vi "CLD 14 Timer Application Solution.vi"() -> ()   [LabVIEW 2009]
doc: "CLD 14 Solution. This is a queued state machine using an array as the queue. The timer was adapted from CLD exercise three.\n\nThe Timer FGV is always running. Use time target equal to zero as the signal the timer is not \"active\""
uses:
  CLD 14 FGV Enum.ctl
  CLD 14 State Machine Enum.ctl
  CLD 14 CSV file enum.ctl
panel:
  out "Time Target (s)":dbl
  out "Elapsed Time (s)":dbl format="%#.2g"
  in  "Stop":bool
  in  "Pause":bool
  in  "cancel":bool
  in  "Start":bool
  in  "Error In":errorcluster
  out "Error Out":errorcluster
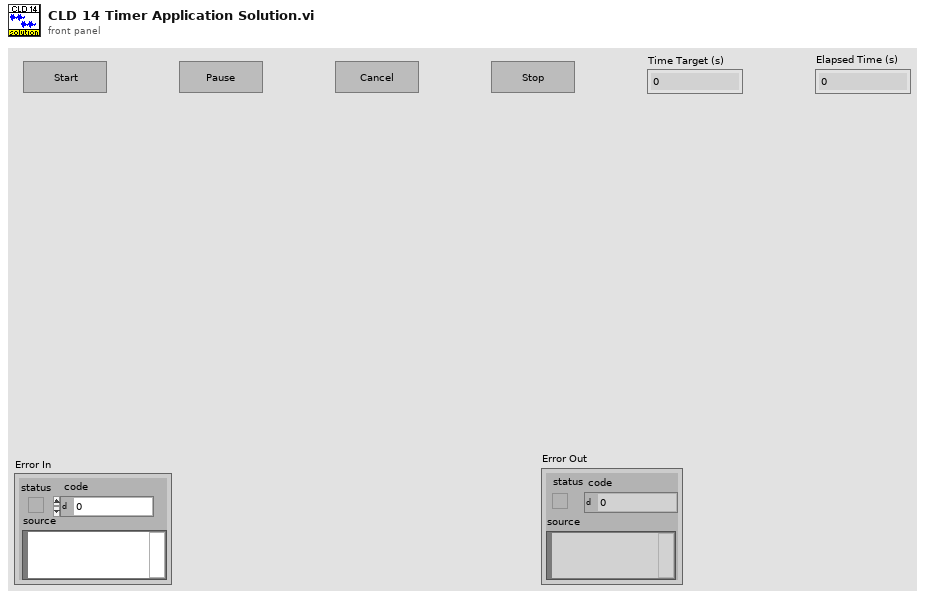
[diagram p1: front panel]
types:
  T1 = typedef "CLD 14 FGV Enum.ctl" = enum16{"Start Timer", "Read Time", "Pause", "UnPause"}
  T2 = typedef "CLD 14 State Machine Enum.ctl" = enum16{"Idle", "Initialize", "Run State", "Change Time", "CheckTime", "Start Time", "Pause", "UnPause"}
  T3 = typedef "CLD 14 CSV file enum.ctl" = enum16{"Read CSV", "Write CSV"}
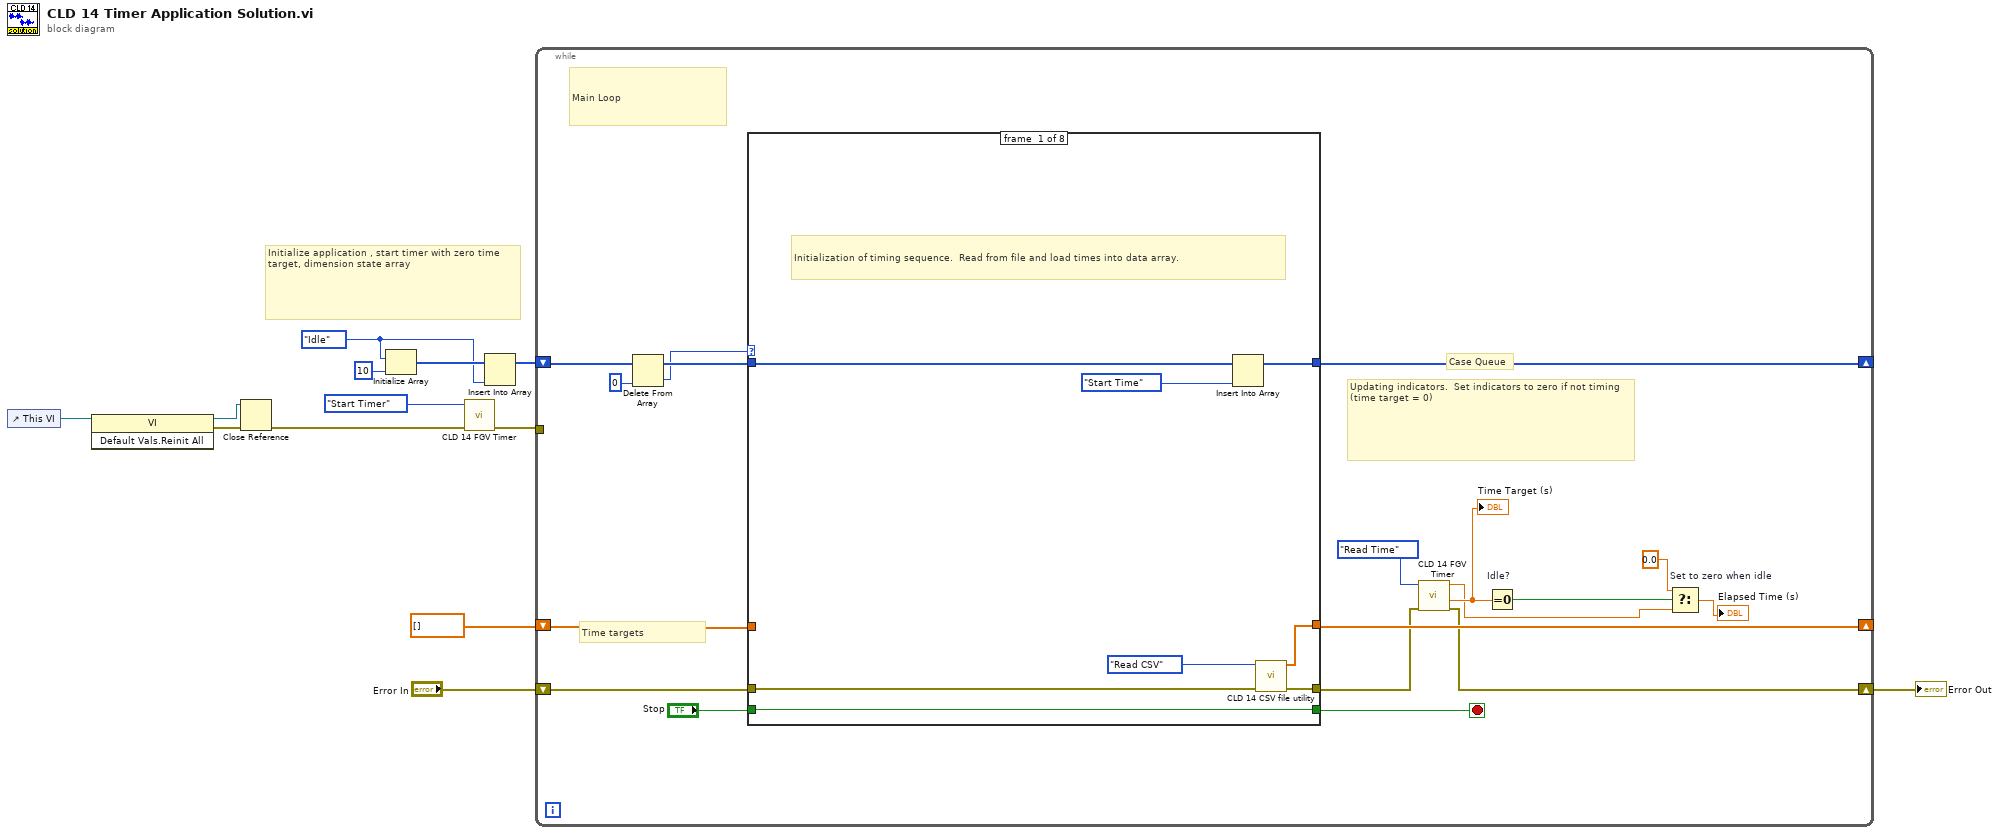
[diagram p0: block diagram]
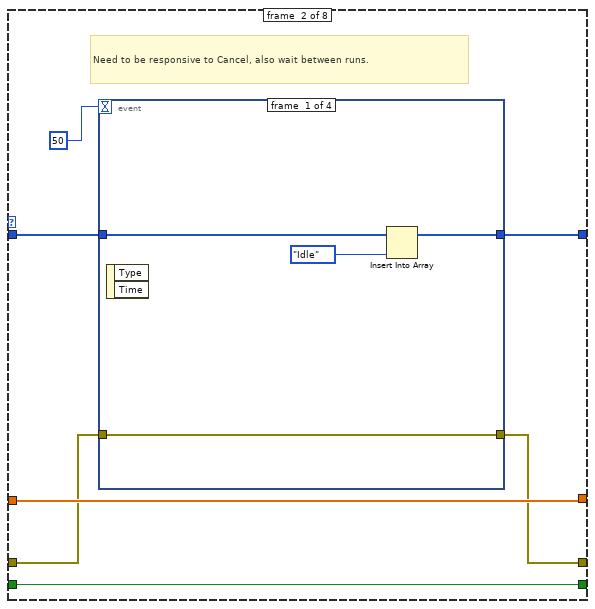
[diagram p2: hidden frame]
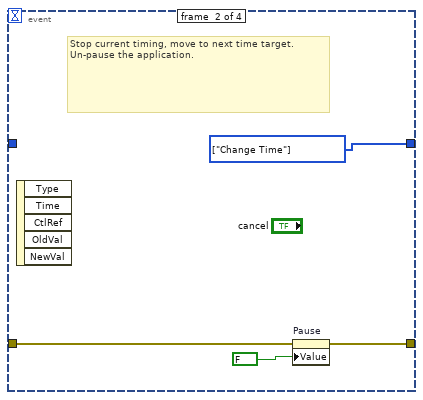
[diagram p3: hidden frame]
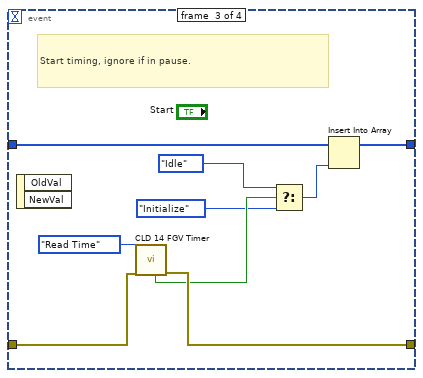
[diagram p4: hidden frame]
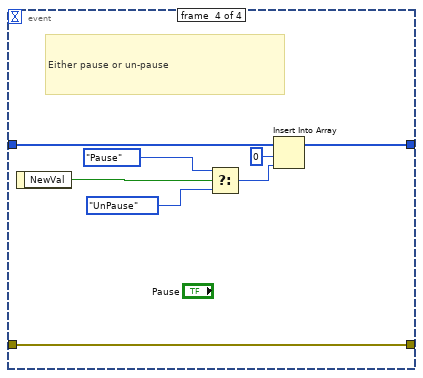
[diagram p5: hidden frame]
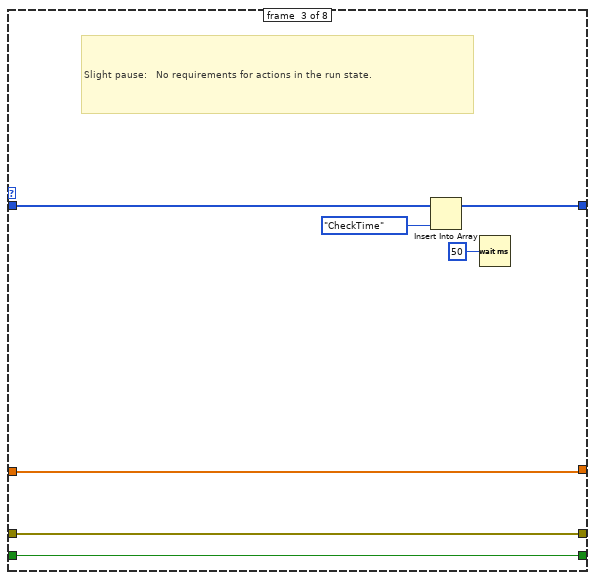
[diagram p6: hidden frame]
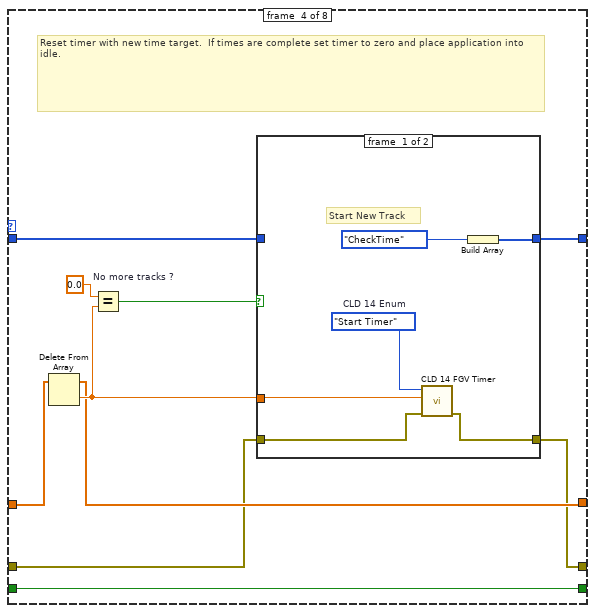
[diagram p7: hidden frame]
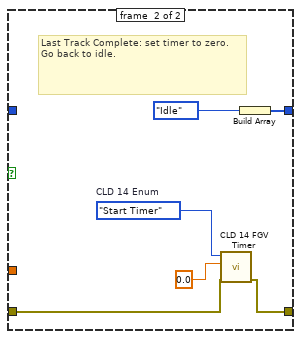
[diagram p8: hidden frame]
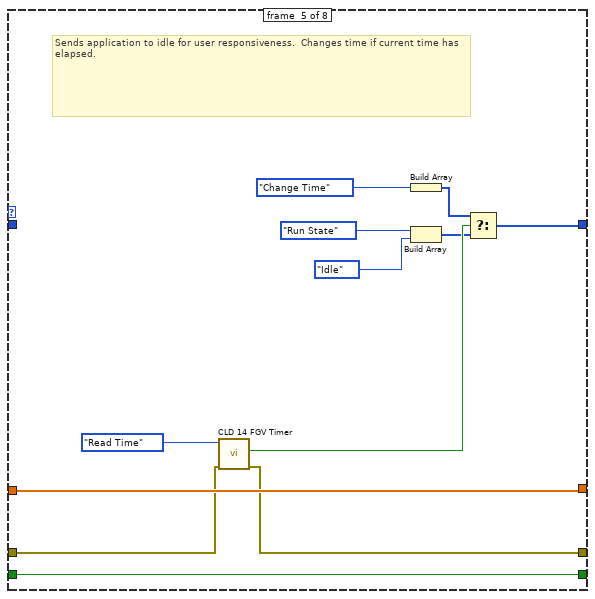
[diagram p9: hidden frame]
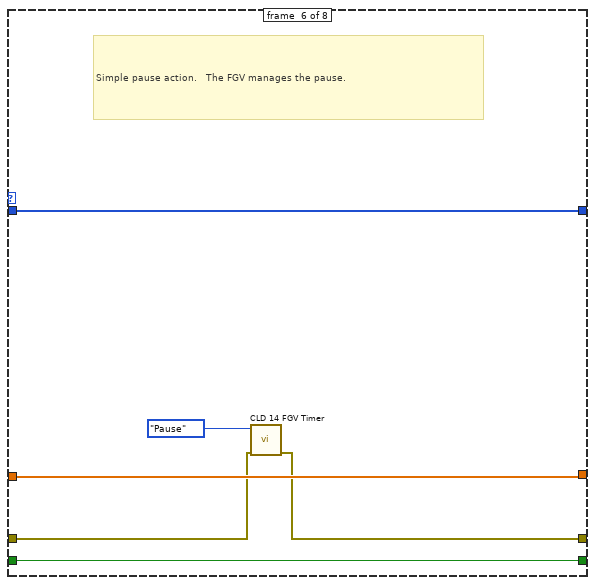
[diagram p10: hidden frame]
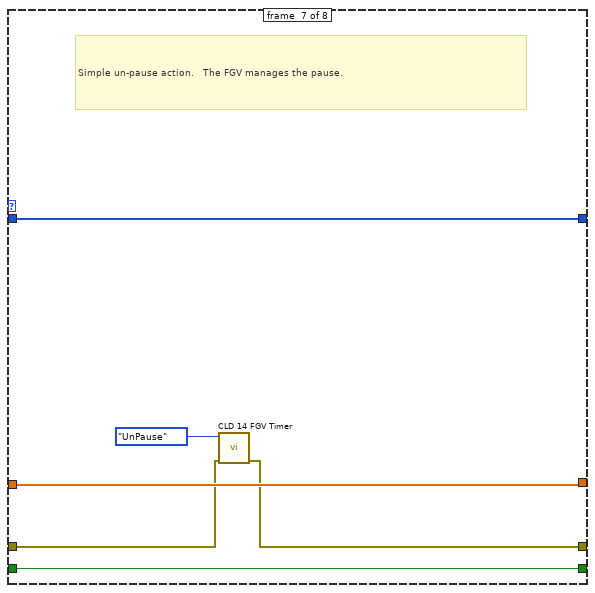
[diagram p11: hidden frame]
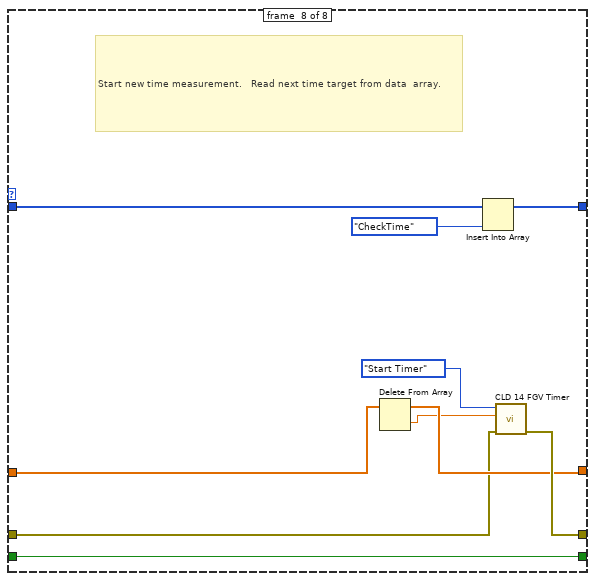
[diagram p12: hidden frame]
diagram:
  w2 = CLD_14_State_Machine_Enum."Idle" ("CLD 14")
  # "Initialize application , start timer with zero time target, dimension state array"
  n1 = control-ref of="This VI"() -> (w8:refnum<vi>)
  n2 = invoke class="VI" method="Default Vals.Reinit All"(reference=w8) -> (reference out=w9:refnum<vi>, error out=w10:errorcluster)  [unwired: 2 in, 1 out]
  n3 = Close Reference(reference=w9, error in (no error)=w10) -> (error out=w7:errorcluster)
  n4 = Initialize Array(w2, 10 ("dimension size")) -> (w4:T2[])
  n5 = call "CLD 14 FGV Timer.vi"("Error In"=w7, "CLD 14 FGV Enum"=CLD_14_FGV_Enum."Start Timer") -> ("Error Out"=w6:errorcluster)  [unwired: 5 in, 4 out]
  n6 = Insert Into Array(array=w4, new element=w2) -> (w3:T2[])  [unwired: 1 in]
  n7 = while {
    shift-right: [w31] -> _
    shift-left: w3 -> [w24]
    shift-right: [w26] -> _
    shift-left: dbl[] [] ("Array") -> [w29]
    tunnel: w6 -> [_]
    shift-right: [w14] -> w12
    shift-left: "Error In" -> [w30]
    stop <- w28 stop-if-true
    # "Case Queue"
    # "Time targets"
    # "Updating indicators.  Set indicators to zero if not timing (time target = 0)"
    # "Main Loop"
    n8 = Delete From Array(array=w24, index=0) -> (deleted portion=w23:T2, array with subset deleted=w25:T2[])  [unwired: 1 in]
    n9 = case shown="\"Start Time\"" w23 {
      tunnel: [w32 w46 w74 w84 w103 w113 w119 w130] -> w31
      tunnel: w30 -> [w39 w42 w78 w80 w109 w115 w121 w127]
      tunnel: [w38 w41 w78 w79 w108 w114 w120 w133] -> w15
      tunnel: [w36 w43 w76 w82 w112 w118 w124 w131] -> w26
      tunnel: w29 -> [_ w43 w76 w83 w112 w118 w124 w132]
      tunnel: "Stop" -> [w35 w45 w77 w88 w111 w117 w123 w134]
      tunnel: [w35 w45 w77 w88 w111 w117 w123 w134] -> w28
      tunnel: w25 -> [w33 w40 w72 w81 _ w113 w119 w128]
      frame #0 {
        # "Initialization of timing sequence.  Read from file and load times into data array."
        n10 = Insert Into Array(array=w33, new element=CLD_14_State_Machine_Enum."Start Time" ("CLD 14")) -> (w32:T2[])  [unwired: 1 in]
        n11 = call "CLD 14 CSV file utility.vi"("Error In"=w39, "CLD 14 Timer Enum"=CLD_14_CSV_file_enum."Read CSV" ("CLD Eighth One Timer Enum")) -> ("Error Out"=w38:errorcluster, "Array"=w36:dbl[])  [unwired: 8 in]
      }
      frame #1 {
        # "Need to be responsive to Cancel, also wait between runs."
        n12 = event shown="[1] \"cancel\": Value Change" {
          selector: _ -> [_ _ _ _]
          dyn-events: _ -> [_ _ _ _]
          timeout: 50 -> [_ _ _ _]
          tunnel: [w49 w54 w63 w69] -> w46
          tunnel: [w50 w51 w59 w71] -> w41
          tunnel: w42 -> [w50 w52 w60 w71]
          tunnel: w40 -> [w47 _ w62 w70]
          event #0 {
            n13 = event-data() -> ()  [unwired: 1 in, 2 out]
            n14 = Insert Into Array(array=w47, new element=CLD_14_State_Machine_Enum."Idle" ("CLD 14")) -> (w49:T2[])  [unwired: 1 in]
          }
          event #1 {
            w54 = T2[] [enum."Change Time"] items=["Idle", "Initialize", "Run State", "Change Time", "CheckTime", "Start Time", "Pause", "UnPause"]
            # "Stop current timing, move to next time target. Un-pause the application."
            n15 = event-data() -> ()  [unwired: 1 in, 5 out]
            n16 = property on="Pause" class="Bool (strict)"(error in=w52, "Value"=FALSE ("Pause")) -> (error out=w51:errorcluster)  [unwired: 1 in, 1 out]
          }
          event #2 {
            # "Start timing, ignore if in pause."
            n17 = event-data() -> ()  [unwired: 1 in, 2 out]
            n18 = call "CLD 14 FGV Timer.vi"("Error In"=w60, "CLD 14 FGV Enum"=CLD_14_FGV_Enum."Read Time" ("CLD 14 Enum")) -> ("Error Out"=w59:errorcluster, "Pause ?"=w58:bool)  [unwired: 5 in, 3 out]
            n19 = Select(t=CLD_14_State_Machine_Enum."Idle" ("CLD 14"), s=w58, f=CLD_14_State_Machine_Enum."Initialize" ("CLD 14")) -> (s? t:f=w55:T2)
            n20 = Insert Into Array(array=w62, new element=w55) -> (w63:T2[])  [unwired: 1 in]
          }
          event #3 {
            # "Either pause or un-pause"
            n21 = event-data() -> ("NewVal"=w68:bool)  [unwired: 1 in]
            n22 = Select(t=CLD_14_State_Machine_Enum."Pause" ("new element/subarray"), s=w68, f=CLD_14_State_Machine_Enum."UnPause" ("new element/subarray")) -> (s? t:f=w65:T2)
            n23 = Insert Into Array(array=w70, index=0, new element=w65) -> (w69:T2[])
          }
        }
      }
      frame #2 {
        # "Slight pause:   No requirements for actions in the run state."
        n24 = Insert Into Array(array=w72, new element=CLD_14_State_Machine_Enum."CheckTime" ("CLD 14")) -> (w74:T2[])  [unwired: 1 in]
        n25 = Wait (ms)(milliseconds to wait=u32 50) -> ()  [unwired: 1 out]
      }
      frame #3 {
        # "Reset timer with new time target.  If times are complete set timer to zero and place application into idle."
        n26 = Delete From Array(array=w83) -> (deleted portion=w85:dbl, array with subset deleted=w82:dbl[])  [unwired: 2 in]
        n27 = Equal? "No more tracks ?"(x=0.0, y=w85) -> (x = y?=w86:bool)
        n28 = case shown="True" w86 {
          tunnel: w85 -> [w94 _]
          tunnel: w80 -> [w93 w98]
          tunnel: [w89 w95] -> w84
          tunnel: w81 -> [_ _]
          tunnel: [w91 w97] -> w79
          frame #0 {
            w92 = CLD_14_FGV_Enum."Start Timer"  # CLD 14 Enum
            # "Start New Track"
            n29 = call "CLD 14 FGV Timer.vi"("Error In"=w93, "Time Target (s) [0]"=w94, "CLD 14 FGV Enum"=w92) -> ("Error Out"=w91:errorcluster)  [unwired: 4 in, 4 out]
            n30 = Build Array(CLD_14_State_Machine_Enum."CheckTime" ("CLD 14")) -> (w89:T2[])
          }
          frame #1 {
            w100 = CLD_14_FGV_Enum."Start Timer"  # CLD 14 Enum
            # "Last Track Complete: set timer to zero.  Go back to idle."
            n31 = call "CLD 14 FGV Timer.vi"("Error In"=w98, "Time Target (s) [0]"=0.0 ("Time Target (s)"), "CLD 14 FGV Enum"=w100) -> ("Error Out"=w97:errorcluster)  [unwired: 4 in, 4 out]
            n32 = Build Array(CLD_14_State_Machine_Enum."Idle" ("CLD 14")) -> (w95:T2[])
          }
        }
      }
      frame #4 {
        # "Sends application to idle for user responsiveness.  Changes time if current time has elapsed."
        n33 = call "CLD 14 FGV Timer.vi"("Error In"=w109, "CLD 14 FGV Enum"=CLD_14_FGV_Enum."Read Time" ("CLD 14 Enum")) -> ("Error Out"=w108:errorcluster, "Has Time Elapsed ?"=w107:bool)  [unwired: 5 in, 3 out]
        n34 = Build Array(CLD_14_State_Machine_Enum."Change Time" ("CLD 14")) -> (w105:T2[])
        n35 = Build Array(CLD_14_State_Machine_Enum."Run State" ("CLD 14"), CLD_14_State_Machine_Enum."Idle" ("CLD 14")) -> (w104:T2[])
        n36 = Select(t=w105, s=w107, f=w104) -> (s? t:f=w103:T2[])
      }
      frame #5 {
        # "Simple pause action.   The FGV manages the pause."
        n37 = call "CLD 14 FGV Timer.vi"("Error In"=w115, "CLD 14 FGV Enum"=CLD_14_FGV_Enum."Pause" ("CLD 14 Enum")) -> ("Error Out"=w114:errorcluster)  [unwired: 5 in, 4 out]
      }
      frame #6 {
        # "Simple un-pause action.   The FGV manages the pause."
        n38 = call "CLD 14 FGV Timer.vi"("Error In"=w121, "CLD 14 FGV Enum"=CLD_14_FGV_Enum."UnPause" ("CLD 14 Enum")) -> ("Error Out"=w120:errorcluster)  [unwired: 5 in, 4 out]
      }
      frame #7 {
        # "Start new time measurement.   Read next time target from data  array."
        n39 = Delete From Array(array=w132) -> (deleted portion=w126:dbl, array with subset deleted=w131:dbl[])  [unwired: 2 in]
        n40 = Insert Into Array(array=w128, new element=CLD_14_State_Machine_Enum."CheckTime" ("CLD 14")) -> (w130:T2[])  [unwired: 1 in]
        n41 = call "CLD 14 FGV Timer.vi"("Error In"=w127, "Time Target (s) [0]"=w126, "CLD 14 FGV Enum"=CLD_14_FGV_Enum."Start Timer" ("CLD 14 Enum")) -> ("Error Out"=w133:errorcluster)  [unwired: 4 in, 4 out]
      }
    }
    n42 = call "CLD 14 FGV Timer.vi"("Error In"=w15, "CLD 14 FGV Enum"=CLD_14_FGV_Enum."Read Time" ("CLD 14 Enum")) -> ("Error Out"=w14:errorcluster, "Time Target Out"=w19:dbl, "Elapsed Time (s.ss)"=w17:dbl)  [unwired: 5 in, 2 out]
    "Time Target (s)" <- w19
    n43 = Equal To 0? "Idle?"(x=w19) -> (x = 0?=w20:bool)
    n44 = Select "Set to zero when idle"(t=0.0, s=w20, f=w17) -> (s? t:f=→"Elapsed Time (s)":dbl)
  }
  "Error Out" <- w12
